vi "Read value.vi"(11 "TestManagerMsg.KVP in":refnum<class "TestManagerMsg.KVP.lvclass">) -> (2 "value":variant, 3 "TestManagerMsg.KVP out":refnum<class "TestManagerMsg.KVP.lvclass">)   [LabVIEW 2013, in "Caraya.lvlib" / "TestManagerMsg.KVP.lvclass"]
uses:
  TestManagerMsg.KVP.lvclass
  TestManagerMsg.KVP.lvclass/TestManagerMsg.KVP.ctl
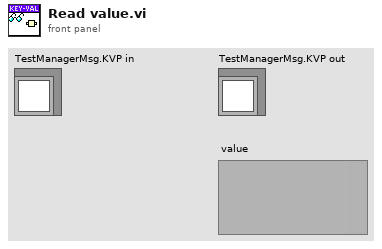
[diagram p1: front panel]
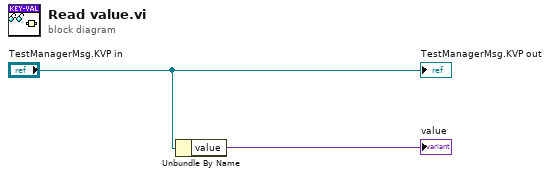
[diagram p0: block diagram]
diagram:
  n1 = Unbundle By Name("TestManagerMsg.KVP in") -> ("value"=→"value":variant)
  "TestManagerMsg.KVP out" <- "TestManagerMsg.KVP in"
